vi "LV SCISDK Get Parameter Integer.vi"(8 "error in (no error)":errorcluster, 10 "handle":u64, 11 "Path":string) -> (0 "error out":errorcluster, 1 "function return":i32, 2 "handle out":u64, 3 "value":i32)   [LabVIEW 2021, in "SciSDK_Labview.lvlib"]
doc: "SCISDKLABVIEW_DLL_API int LV_SCISDK_GetParameterInteger(char* Path, int* value, void* handle);"
uses:
  SciSDK_Labview.lvlib
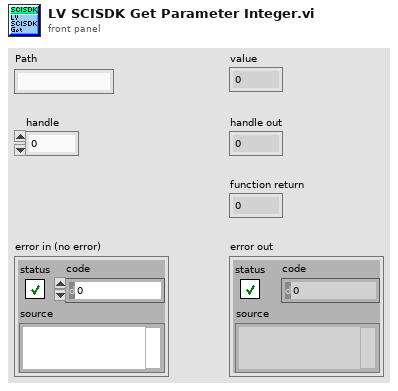
[diagram p1: front panel]
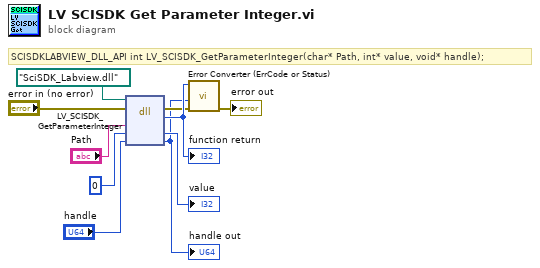
[diagram p0: block diagram]
diagram:
  # "SCISDKLABVIEW_DLL_API int LV_SCISDK_GetParameterInteger(char* Path, int* value, void* handle);"
  n1 = dll-call lib="C:/git/scisdk/SciSDK_VC++/x64/Debug/SciSDK_Labview.*" fn="LV_SCISDK_GetParameterInteger"(path in=path "SciSDK_Labview.dll", error in="error in (no error)", "Path"="Path", "value"=0, "handle"="handle") -> (error out=w4:errorcluster, "return type"=w10:i32, "value"=→"value":i32, "handle"=w1:u64)  [unwired: 2 in, 1 out]
  "function return" <- w10
  "handle out" <- w1
  n2 = call "Error Converter (ErrCode or Status).vi"("error in (no error)"=w4, "handle"=w1, "error code"=w10) -> ("error out"=→"error out":errorcluster)  [unwired: 8 in]
